vi "Info.vi"(8 "error in (no error)":errorcluster, 11 "Channel BOOL in":refnum<class "Channel BOOL.lvclass">) -> (0 "error out":errorcluster, 2 "Info":T1, 3 "Channel BOOL out":refnum<class "Channel BOOL.lvclass">)   [LabVIEW 2020, in "Vecto.lvlib" / "Channel BOOL.lvclass"]
uses:
  Channel BOOL.lvclass
  Channel BOOL.lvclass/Channel BOOL.ctl
  Group/Group.lvclass
  Group BOOL/Group BOOL.lvclass
  C:/dev/lv20CE/relink/lv-vecto/Vecto/Group/Group.lvclass
  C:/dev/lv20CE/relink/lv-vecto/Vecto/Group BOOL/Group BOOL.lvclass
  Channel Info.ctl
  VectoConfig/VectoConfig.lvlib
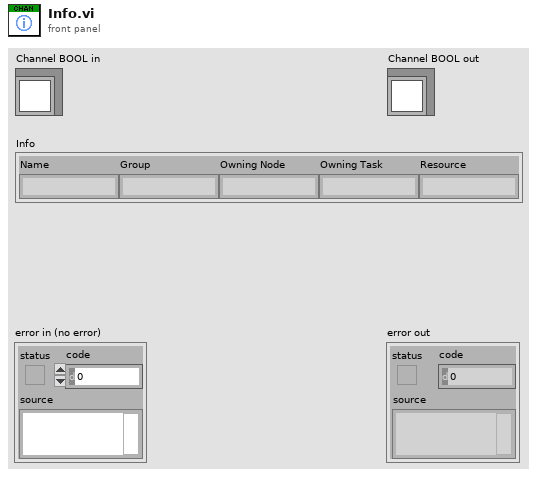
[diagram p1: front panel]
types:
  T1 = typedef "VectoConfig.lvlib/Channel Info.ctl" = cluster{"Name":string, "Group":string, "Owning Node":string, "Owning Task":string, "Resource":string}
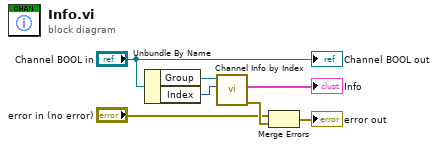
[diagram p0: block diagram]
diagram:
  n1 = Unbundle By Name("Channel BOOL in") -> ("Group"=w7:refnum<class "Group BOOL.lvclass">, "Index"=w5:i32)
  n2 = call "Channel Info by Index.vi"("Index"=w5, "Group in"=w7) -> ("error out"=w6:errorcluster, "Channel Info"=→"Info":T1)  [unwired: 7 in, 1 out]
  n3 = Merge Errors("error in (no error)", w6) -> (→"error out":errorcluster)
  "Channel BOOL out" <- "Channel BOOL in"
